vi "Get VI Metrics - Simple VI - Returns Correct Numbers.vi"() -> ()   [LabVIEW 2017, in "Cobertura.Tests.lvlib" / "Code Inspector.lvlib"]
uses:
  Code Inspector.lvlib
  Simple VI.vi
  Cobertura/Code Inspector/Code Inspector.lvclass
  <vilib>/PNR/Transparent Assertions/Transparent Assertions/Transparent Assertions.lvlib
panel:
  out "error out":errorcluster
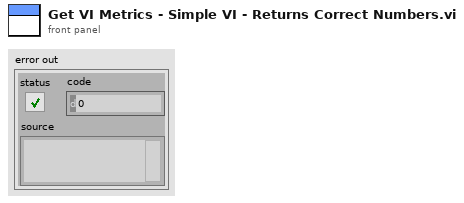
[diagram p1: front panel]
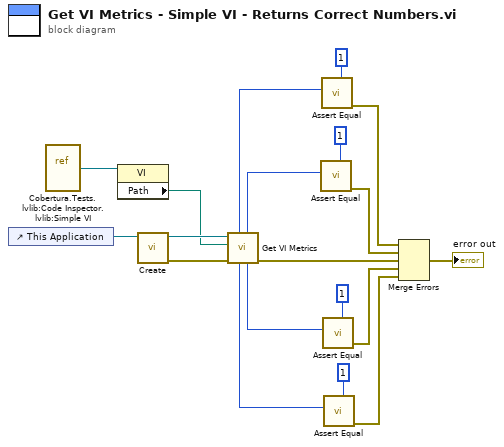
[diagram p0: block diagram]
diagram:
  n1 = control-ref of="This Application"() -> (w17:refnum<vi>)
  n2 = vi-ref "Cobertura.Tests.lvlib:Code Inspector.lvlib:Simple VI.vi"() -> (w16:refnum<vi>)
  n3 = property class="VI"(reference=w16) -> ("Path"=w15:path)  [unwired: 1 in, 2 out]
  n4 = call "Create.vi"("Application"=w17) -> ("error out"=w18:errorcluster, "Code Inspector"=w19:refnum<class "Code Inspector.lvclass">)  [unwired: 9 in]
  n5 = call-dynamic "Get VI Metrics.vi"("error in (no error)"=w18, "VI Path"=w15, "Code Inspector in"=w19) -> ("error out"=w6:errorcluster, "Total Diagram Count"=w10:i32, "Total Node Count"=w14:i32, "Uncovered Diagram Count"=w9:i32, "Uncovered Node Count"=w13:i32)  [unwired: 2 in, 2 out]
  n6 = call <vilib>:"Assert Equal.vi"("Expected"=1, "Actual"=w14) -> ("error out"=w5:errorcluster)  [unwired: 9 in]
  n7 = call <vilib>:"Assert Equal.vi"("Expected"=1, "Actual"=w13) -> ("error out"=w4:errorcluster)  [unwired: 9 in]
  n8 = call <vilib>:"Assert Equal.vi"("Expected"=1, "Actual"=w10) -> ("error out"=w3:errorcluster)  [unwired: 9 in]
  n9 = call <vilib>:"Assert Equal.vi"("Expected"=1, "Actual"=w9) -> ("error out"=w2:errorcluster)  [unwired: 9 in]
  n10 = Merge Errors(w4, w5, w6, w3, w2) -> (→"error out":errorcluster)
